vi "WGN_Query.vi"(0 "System no.":i32=1 min=1 max=4 step=1, 2 "Generator ID":string[](array[string]), 3 "All IDs?":bool, 4 "identifier?":bool=TRUE, 5 "error in":errorcluster) -> (14 "No. of Cycles":i32[](array[numeric]), 19 "error out":errorcluster)   [LabVIEW 2020]
doc: "Returns the number of finished wave cycles since last WGO. Only starting a wave generator by sending the corresponding WGO command resets the counter to 0. The counter is halted (but not resetted) if the wave generator is stopped by sending the corresponding WGO or #24 command or by a hardware trigger. A counter overflow does not set any error. The counter overflow value depends on the hardware, for details see user manual.\n\nE-709: If All IDs? = TRUE, Identifier must be FALSE."
panel:
  # "Returns the number of finished wave cycles since last WGO."
  # "If all IDs: use"
  # "Query"
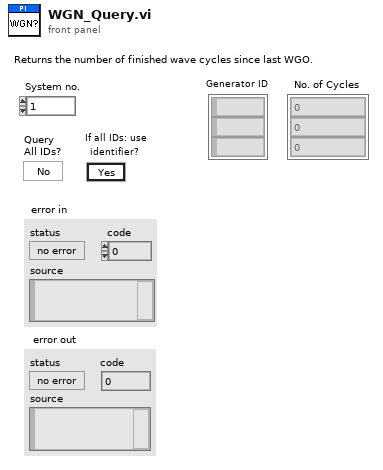
[diagram p1: front panel]
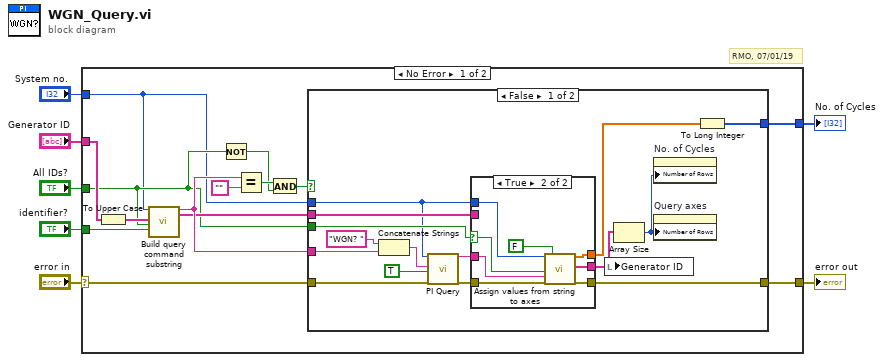
[diagram p0: block diagram]
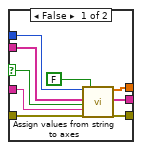
[diagram p2: hidden frame]
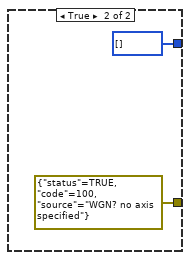
[diagram p3: hidden frame]
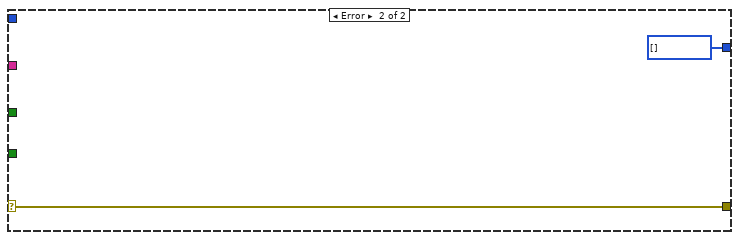
[diagram p4: hidden frame]
diagram:
  # "RMO, 07/01/19"
  n1 = case shown="No Error" "error in" {
    selector: "error in" -> [w10 w56]
    tunnel: [w11 i32[] [] ("Values")] -> w7
    tunnel: "Generator ID" -> [w21 _]
    tunnel: [w9 w56] -> w5
    tunnel: "identifier?" -> [w18 _]
    tunnel: "System no." -> [w12 _]
    tunnel: "All IDs?" -> [w13 _]
    frame No Error {
      n2 = To Upper Case(1:w21) -> (0:w19:string[])
      n3 = call "Build query command substring.vi"("System no."=w12, "Axes to query in"=w19, "Query\nAll axes?"=w13, "For all axes: use\nAxis identifier?"=w18) -> ("Command substring"=w17:string, "Axes to query out"=w14:string[])  [unwired: 2 in, 12 out]
      n4 = Not(x=w13) -> (.not. x?=w15:bool)
      n5 = Equal?(x=w17, y="" ("x")) -> (x = y?=w16:bool)
      n6 = And(x=w16, y=w15) -> (x .and. y?=w8:bool)
      n7 = case shown="False" w8 {
        tunnel: w17 -> [w33 _]
        tunnel: w14 -> [w32 _]
        tunnel: w13 -> [w30 _]
        tunnel: w12 -> [w29 _]
        tunnel: [w26 i32[] []] -> w11
        tunnel: w10 -> [w25 _]
        tunnel: [w24 errorcluster {"status"=TRUE, "code"=100, "source"="WGN? no axis specified"} ("error out")] -> w9
        frame False {
          n8 = Concatenate Strings("WGN? ", w33) -> (w34:string)
          n9 = call "PI Query.vi"("System no."=w29, "String to send"=w34, "Attach termination char.?"=TRUE ("Attach Linefeed?"), "error in"=w25) -> ("String read"=w22:string, "error out"=w23:errorcluster)  [unwired: 3 in, 11 out]
          n10 = case shown="True" w30 {
            selector: w30 -> [w39 w49]
            tunnel: [w45 w48] -> w31
            tunnel: w29 -> [w44 w53]
            tunnel: w32 -> [w43 _]
            tunnel: w22 -> [w42 w52]
            tunnel: [w41 w51] -> w24
            tunnel: w23 -> [w40 w50]
            tunnel: [w38 w47] -> w27
            frame False {
              n11 = call "Assign values from string to axes.vi"("System no."=w44, "Queried axes"=w43, "All axes queried?"=w39, "Input String"=w42, "error in"=w40, "Axes related?"=FALSE) -> ("Values"=w45:dbl[], "Queried axes out"=w38:string[], "error out"=w41:errorcluster)  [unwired: 3 in, 8 out]
            }
            frame True {
              n12 = call "Assign values from string to axes.vi"("System no."=w53, "All axes queried?"=w49, "Input String"=w52, "error in"=w50, "Axes related?"=FALSE) -> ("Values"=w48:dbl[], "Queried axes out"=w47:string[], "error out"=w51:errorcluster)  [unwired: 4 in, 8 out]
            }
          }
          n13 = local write "Generator ID"(w27) -> ()
          n14 = Array Size(array=w27) -> (size(s)=w28:i32)
          n15 = property on="No. of Cycles" class="Arr (strict)"("Number of Rows"=w28) -> ()  [unwired: 2 in, 2 out]
          n16 = property on="Query axes" class="Arr (strict)"("Number of Rows"=w28) -> ()  [unwired: 2 in, 2 out]
          n17 = To Long Integer(number=w31) -> (32bit integer=w26:i32[])
        }
        frame True {
        }
      }
    }
    frame Error {
    }
  }
  "error out" <- w5
  "No. of Cycles" <- w7
